vi "Val Change.vi"(11 "data":variant) -> (3 "Boolean":bool)   [LabVIEW 2015]
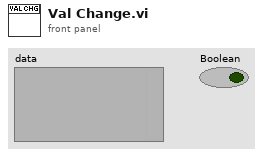
[diagram p1: front panel]
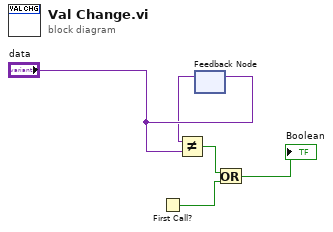
[diagram p0: block diagram]
diagram:
  n1 = First Call?() -> (First Call?: T/F=w3:bool)
  n2 = feedback #1() -> (w1:variant)  [unwired: 1 in]
  n3 = Not Equal?(x=w1, y="data") -> (x != y?=w2:bool)
  n4 = feedback-in #1("data") -> ()
  n5 = Or(x=w2, y=w3) -> (x .or. y?=→"Boolean":bool)
